vi "setFPGAReference.vi"(10 "FPGAReference":refnum<k20>, 11 "MyHealthAndStatusReadFIFO in":refnum<class "DisplacementTimestampFIFO.lvclass">) -> (3 "MyHealthAndStatusReadFIFO out":refnum<class "DisplacementTimestampFIFO.lvclass">)   [LabVIEW 2016, in "DisplacementTimestampFIFO.lvclass"]
uses:
  DisplacementTimestampFIFO.lvclass
  DisplacementTimestampFIFO.lvclass/DisplacementTimestampFIFO.ctl
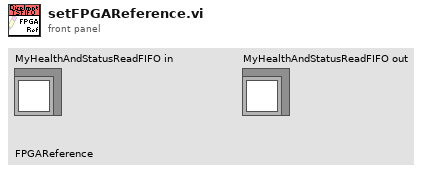
[diagram p1: front panel]
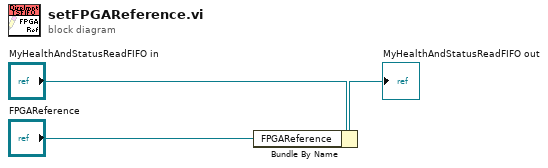
[diagram p0: block diagram]
diagram:
  n1 = Bundle By Name(cluster="MyHealthAndStatusReadFIFO in", "FPGAReference"="FPGAReference") -> (→"MyHealthAndStatusReadFIFO out":refnum<class "DisplacementTimestampFIFO.lvclass">)
